vi "p2.vi"() -> ()   [LabVIEW 2025, in "d6.lvlib"]
uses:
  d6.lvlib
  lv2025-aoc/AOC/AOC.lvlib
  <userlib>/_OpenG.lib/string/string.llb/openg_string.lvlib
panel:
  in  "Example":string="123 328  51 64 \n 45 64  387 23 \n  6 98  215 314\n*   +   *   +  "
  in  "Example 2":bool=TRUE
  out "Answer":u64=1909
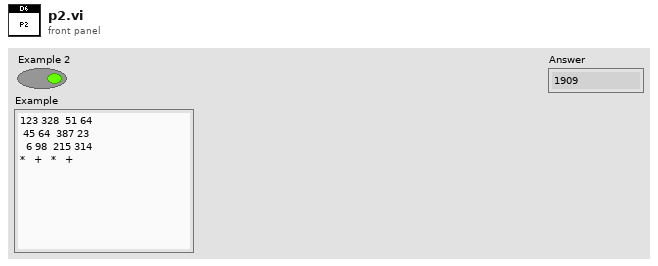
[diagram p1: front panel]
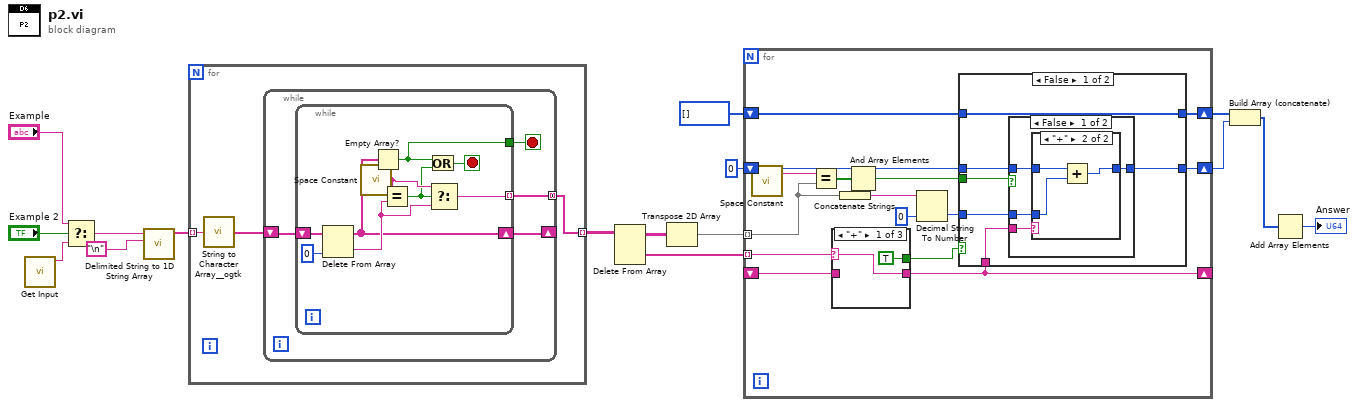
[diagram p0: block diagram]
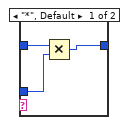
[diagram p2: hidden frame]
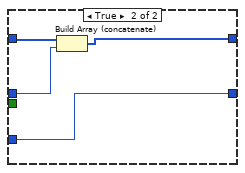
[diagram p4: hidden frame]
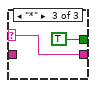
[diagram p6: hidden frame]
diagram:
  n1 = call "Get Input.vi"() -> ("Input"=w16:string)  [unwired: 11 in]
  n2 = Select(t="Example", s="Example 2", f=w16) -> (s? t:f=w9:string)
  n3 = call <vilib>:"Delimited String to 1D String Array.vi"("delimiter"="\n", "delimited string"=w9) -> ("string array"=w11:string[])  [unwired: 9 in]
  n4 = for {
    tunnel: w11 -> [w19] mode=indexing
    tunnel: [w17] -> w10 mode=indexing
    n5 = call <userlib>:"String to Character Array__ogtk.vi"("Input String"=w19) -> ("Character Array"=w18:string[])
    n6 = while {
      tunnel: [w21] -> w17 mode=concatenating
      shift-right: [w22] -> _
      shift-left: w18 -> [w23]
      stop <- w20 stop-if-true
      n7 = while {
        shift-right: [w26] -> w22
        shift-left: w23 -> [w32]
        tunnel: [w27] -> w21 mode=indexing
        tunnel: [w25] -> w20
        stop <- w24 stop-if-true
        n8 = Delete From Array(array=w32, index=0) -> (deleted portion=w28:string, array with subset deleted=w26:string[])  [unwired: 1 in]
        n9 = call <vilib>:"Space Constant.vi"() -> ("String"=w31:string)
        n10 = Empty Array?(array=w26) -> (empty?=w25:bool)
        n11 = Equal?(x=w31, y=w28) -> (x = y?=w30:bool)
        n12 = Or(x=w25, y=w30) -> (x .or. y?=w24:bool)
        n13 = Select(t=w31, s=w30, f=w28) -> (s? t:f=w27:string)
      }
    }
  }
  n14 = Delete From Array(array=w10) -> (deleted portion=w7:string[], array with subset deleted=w8:string[][])  [unwired: 3 in]
  n15 = Transpose 2D Array(2D array=w8) -> (transposed array=w6:string[][])
  n16 = for {
    tunnel: w6 -> [w36] mode=indexing
    tunnel: w7 -> [w47] mode=indexing
    shift-right: [w43] -> _
    shift-left: _ -> [w45]
    shift-right: [w41] -> w1
    shift-left: u64 0 -> [w40]
    shift-right: [w37] -> w3
    shift-left: u64[] [] -> [w38]
    n17 = call <vilib>:"Space Constant.vi"() -> ("String"=w35:string)
    n18 = Equal?(x=w35, y=w36) -> (x = y?=w34:bool[])
    n19 = case shown="\"+\"" w47 {
      selector: w47 -> [w70 _ w73]
      tunnel: [w70 w71 w73] -> w43
      tunnel: w45 -> [_ w71 _]
      tunnel: [TRUE _ TRUE] -> w42
      frame "+" {
      }
      frame Default {
      }
      frame "*" {
      }
    }
    n20 = Concatenate Strings(w36) -> (w46:string)
    n21 = And Array Elements(Boolean array=w34) -> (logical AND=w33:bool)
    n22 = Decimal String To Number(string=w46, default (0L)=u64 0 ("default (0 I32)")) -> (number=w44:u64)  [unwired: 1 in, 1 out]
    n23 = case shown="False" w42 {
      tunnel: w44 -> [w53 w68]
      tunnel: w43 -> [w52 _]
      tunnel: [w49 w68] -> w41
      tunnel: w40 -> [w50 w66]
      tunnel: w38 -> [w51 w67]
      tunnel: [w51 w65] -> w37
      tunnel: w33 -> [w48 _]
      frame False {
        n24 = case shown="False" w48 {
          tunnel: w53 -> [w57 _]
          tunnel: w52 -> [w56 _]
          tunnel: w50 -> [w55 w64]
          tunnel: [w54 w64] -> w49
          frame False {
            n25 = case shown="\"+\"" w56 {
              tunnel: w57 -> [w59 w62]
              tunnel: w55 -> [w60 w63]
              tunnel: [w58 w61] -> w54
              frame "*", Default {
                n26 = Multiply(x=w60, y=w59) -> (x*y=w58:u64)
              }
              frame "+" {
                n27 = Add(x=w63, y=w62) -> (x+y=w61:u64)
              }
            }
          }
          frame True {
          }
        }
      }
      frame True {
        n28 = Build Array (concatenate)(w67, w66) -> (w65:u64[])
      }
    }
  }
  n29 = Build Array (concatenate)(w3, w1) -> (w2:u64[])
  n30 = Add Array Elements(numeric array=w2) -> (sum=→"Answer":u64)
